vi "Get Optimiser Parameters - Numeric.vi"(8 "error in (no error)":errorcluster, 11 "Optimiser Cell in":refnum<class "Optimiser Cell.lvclass">) -> (0 "error out":errorcluster, 2 "Parameters - Numeric":T1[](array[typedef]), 3 "Optimiser Cell out":refnum<class "Optimiser Cell.lvclass">)   [LabVIEW 2020, in "CIRCUS_uServices.lvlib" / "Run Utilities.lvlib" / "Optimiser Cell.lvclass"]
uses:
  Optimiser Cell.lvclass
  Optimise parameter - numeric.ctl
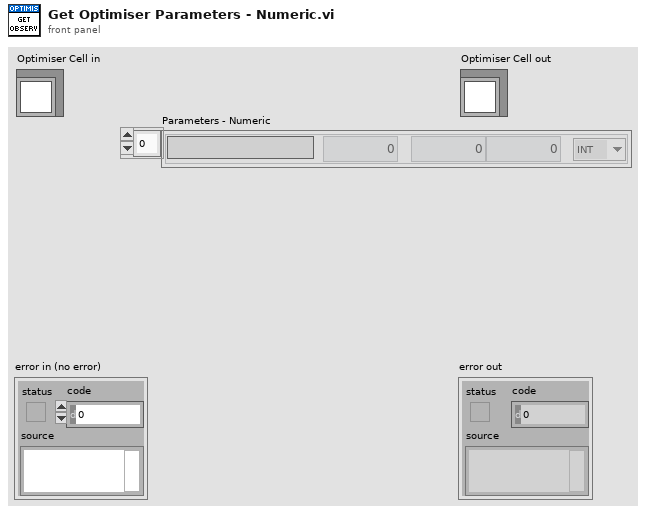
[diagram p1: front panel]
types:
  T1 = typedef "CIRCUS_uServices.lvlib/Run Utilities.lvlib/Optimiser Cell.lvclass/Optimise parameter - numeric.ctl" = cluster{"Name":string, "Start value":dbl, "From":dbl, "To":dbl, "dtype":enum16{"INT", "DBL"}}
  T2 = typedef "Run Utilities.lvlib/Optimiser Cell.lvclass/Optimise parameter - numeric.ctl" = cluster{"Name":string, "Start value":dbl, "From":dbl, "To":dbl, "dtype":enum16{"INT", "DBL"}}
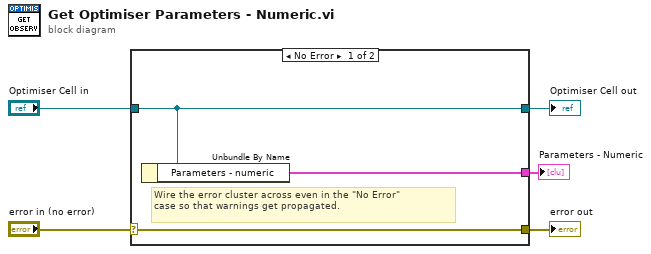
[diagram p0: block diagram]
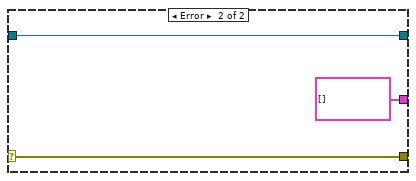
[diagram p2: hidden frame]
diagram:
  n1 = case shown="No Error" "error in (no error)" {
    selector: "error in (no error)" -> [w8 w11]
    tunnel: [w8 w11] -> w4
    tunnel: [w7 w10] -> w2
    tunnel: "Optimiser Cell in" -> [w7 w10]
    tunnel: [w6 T1[] [] ("Accessors:Parameters - Numeric")] -> w1
    frame No Error {
      # "Wire the error cluster across even in the \"No Error\"\ncase so that warnings get propagated."
      n2 = Unbundle By Name(w7) -> ("Parameters - numeric"=w6:T2[])
    }
    frame Error {
    }
  }
  "error out" <- w4
  "Optimiser Cell out" <- w2
  "Parameters - Numeric" <- w1
